vi "Write Logged_On.vi"(8 "error in":errorcluster, 10 "Logged_On":bool, 11 "Base Software in":refnum<class "Main.lvclass">) -> (0 "error out":errorcluster, 3 "Base Software out":refnum<class "Main.lvclass">)   [LabVIEW 2023, in "Main.lvlib" / "Main.lvclass"]
uses:
  Project/Main.lvclass
  Project/Main.lvclass/Main.ctl
  builds/Engine/Engine.lvlibp/Custom Controls/System Status.ctl
  builds/Engine/Engine.lvlibp/Project/Engine.lvclass
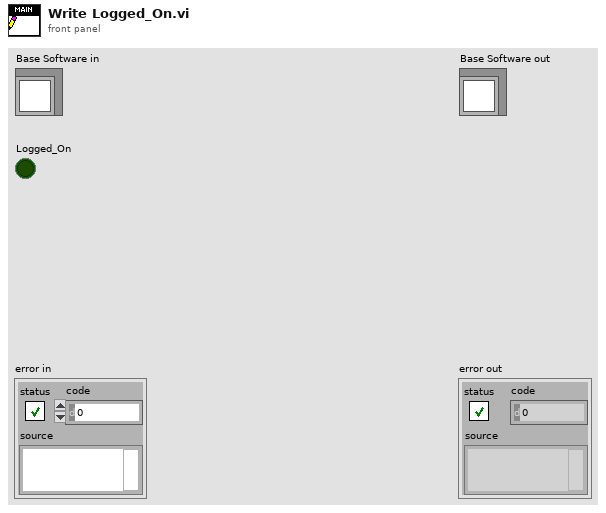
[diagram p1: front panel]
types:
  T1 = typedef "Engine.lvlibp/Engine.lvclass/System Status.ctl" = enum16{"Logged Off", "UUT_Info_Missing", "Idle", "Error", "Warning", "Loading", "Config", "Manual", "Automation", "Report_View", "Previous"}
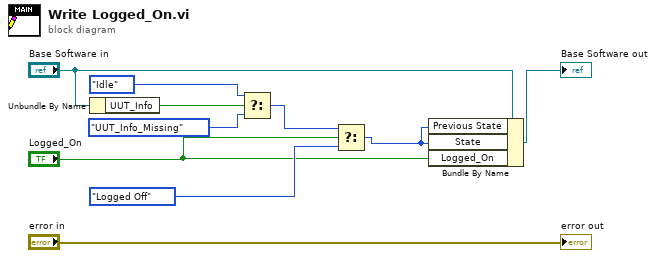
[diagram p0: block diagram]
diagram:
  n1 = Unbundle By Name("Base Software in") -> ("UUT_Info"=w5:bool)
  n2 = Select(t=System_Status."Idle" ("State"), s=w5, f=System_Status."UUT_Info_Missing" ("State")) -> (s? t:f=w2:T1)
  n3 = Select(t=w2, s="Logged_On", f=System_Status."Logged Off" ("State")) -> (s? t:f=w1:T1)
  n4 = Bundle By Name(cluster="Base Software in", "Previous State"=w1, "State"=w1, "Logged_On"="Logged_On") -> (→"Base Software out":refnum<class "Main.lvclass">)
  "error out" <- "error in"
